vi "RF_Rsrc.vi"(7 "RF":T1 items=["RF_0", "RF_1", "RF_2", "RF_3"], 8 "Error_In":errorcluster, 10 "K7_1":refnum<visa-resource-name>, 11 "K7_0":refnum<visa-resource-name>) -> (0 "Error_Out":errorcluster, 3 "Rsrc":refnum<visa-resource-name>)   [LabVIEW 2018]
uses:
  Types/RF.ctl
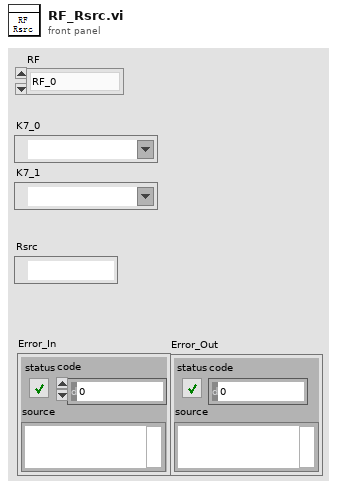
[diagram p1: front panel]
types:
  T1 = typedef "RF.ctl" = u16
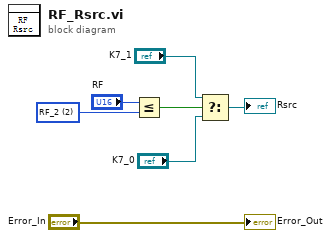
[diagram p0: block diagram]
diagram:
  w6 = T1 2 items=["RF_0", "RF_1", "RF_2", "RF_3"] ("y")
  n1 = Less Or Equal?(x="RF", y=w6) -> (x <= y?=w5:bool)
  n2 = Select(t="K7_1", s=w5, f="K7_0") -> (s? t:f=→"Rsrc":refnum<visa-resource-name>)
  "Error_Out" <- "Error_In"
